vi "ExTestKineticsVClk.vi"() -> ()   [LabVIEW 2010]
panel:
  out "Max Vertical Clock":u32
  out "Min Vertical Clock":u32
  out "Vertical Clock":u32
  in  "Vertical Clock":u32=2 min=1 max=16 step=1
  in  "Enum":T1(ring)
  in  "Window Size":u32=10 min=1 step=1
  out "Boolean":bool
  out "x Size":u32
  out "x post":u32
  out "x pre":u32
  out "y Size":u32
  out "y post":u32
  out "y pre":u32
  in  "Software Accumulation":u32=1 min=1 step=1
  in  "Intensifier":bool
  in  "Temperature":dbl=-10.0 format="%.2f"
  in  "Exposure":dbl min=0.0 step=1e-06 format="%.5f"
  in  "stop":bool
  in  "Store":bool
  out "error out":errorcluster
  in  "error in (no error)":errorcluster
  # "ExCircularBufBin2x:\nThis example only works with cameras with circualar \nbuffer capability. This routine will continously display an\nimage binned by 2 in both the x and the y direction. It \nwill store in append mode the frames while \nthe store toggle switch is on."
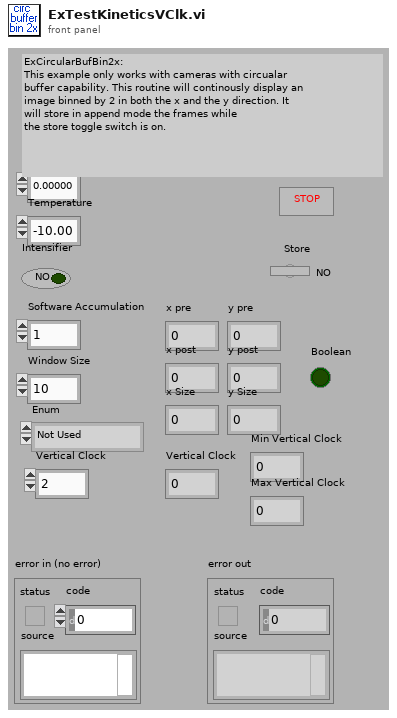
[diagram p1: front panel]
types:
  T1 = enum32{"Not Used", "No Trigger", "Single Trigger", "Multiple Trigger"}
  T2 = cluster{"Param ID":u32, "Avail Flag":u8, "Current Value":dbl, "Default Value":dbl, "Min Value":dbl, "Max Value":dbl, "Increment":dbl, "Data Type":u32, "Access Type":u32, "Bit Used Flag":u32, "Number of Enums":u32, "Description":string}
  T3 = cluster{"Pre Y":u32, "Post Y":u32, "Parallel (Y) Size":u32, "Pre X":u32, "Post X":u32, "Serial (X) Size":u32}
  T4 = cluster{"Camera Handle":u32, "Pulser Handle":u32, "File Handle":u32, "Display Handle":u32, "Image Handle":u32}
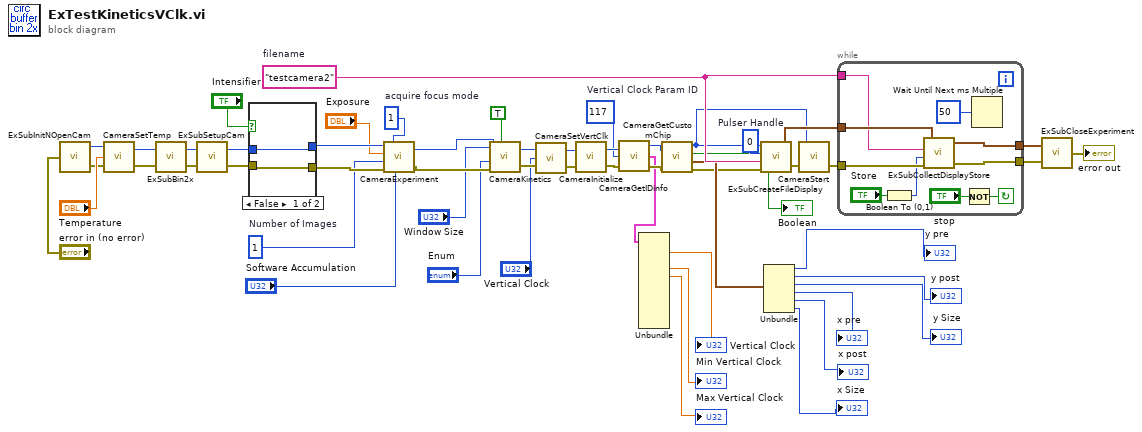
[diagram p0: block diagram]
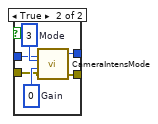
[diagram p2: hidden frame]
diagram:
  w5 = 117  # Vertical Clock Param ID
  w45 = u32 0  # Pulser Handle
  w21 = u32 1  # acquire focus mode
  w23 = u32 1  # Number of Images
  w54 = "testcamera2"  # filename
  n1 = call "ExSubInitNOpenCam.vi"("error in (no error)"="error in (no error)") -> ("Camera Handle"=w43:u32, "error out"=w41:errorcluster)
  n2 = call <userlib>:"CameraSetTemp.vi"("error in (no error)"=w41, "Temperature"="Temperature", "Camera Handle"=w43) -> ("error out"=w29:errorcluster, "Camera Handle"=w30:u32)
  n3 = call "ExSubBin2x.vi"("error in (no error)"=w29, "Camera Handle"=w30) -> ("error out"=w40:errorcluster, "Camera Handle"=w46:u32)
  n4 = call "ExSubSetupCam.vi"("error in (no error)"=w40, "Camera Handle"=w46) -> ("error out"=w27:errorcluster, "Camera Handle"=w28:u32)
  n5 = case shown="False" "Intensifier" {
    tunnel: [w56 w62] -> w26
    tunnel: [w55 w61] -> w25
    tunnel: w28 -> [w56 w58]
    tunnel: w27 -> [w55 w57]
    frame False {
    }
    frame True {
      w59 = u32 0  # Gain
      w60 = u32 3  # Mode
      n6 = call <userlib>:"CameraIntensMode.vi"("error in"=w57, "Intensifier Gain"=w59, "Mode"=w60, "Camera Handle"=w58) -> ("error out"=w61:errorcluster, "Camera Handle"=w62:u32)
    }
  }
  n7 = call <userlib>:"CameraExperiment.vi"("Number of Accumulations"="Software Accumulation", "Acquire / Focus Flag"=w21, "error in"=w25, "Number of Images"=w23, "Exposure (sec)"="Exposure", "Camera Handle"=w26) -> ("error out"=w19:errorcluster, "Camera Handle"=w20:u32)
  n8 = call <userlib>:"CameraKinetics.vi"("Camera Handle"=w20, "Window Size"="Window Size", "TriggerMode"="Enum", "error in (no error)"=w19, "Enable/Disable Kinetics"=TRUE) -> ("Camera Handle"=w13:u32, "error out"=w14:errorcluster)
  n9 = call <userlib>:"CameraSetVertClk.vi"("error in (no error)"=w14, "Vertical Clock"="Vertical Clock", "Camera Handle"=w13) -> ("error out"=w11:errorcluster, "Camera Handle"=w10:u32)
  n10 = call <userlib>:"CameraInitialize.vi"("error in"=w11, "Camera Handle"=w10) -> ("error out"=w9:errorcluster, "Camera Handle"=w6:u32)
  n11 = call <userlib>:"CameraGetIDinfo.vi"("error in"=w9, "Param ID"=w5, "Camera handle"=w6) -> ("error out"=w8:errorcluster, "Param ID Information"=w4:T2, "Camera handle"=w7:u32)
  n12 = Unbundle(w4) -> ("Current Value"=→"Vertical Clock":dbl, "Min Value"=→"Min Vertical Clock":dbl, "Max Value"=→"Max Vertical Clock":dbl)  [unwired: 9 out]
  n13 = call <userlib>:"CameraGetCustomChip.vi"("Camera Handle"=w7, "error in (no error)"=w8) -> ("Camera Handle"=w16:u32, "Custum chip Enable/Disable status"=→"Boolean":bool, "CameraGetCustomChip"=w39:T3, "error out"=w32:errorcluster)
  n14 = call "ExSubCreateFileDisplay.vi"("error in (no error)"=w32, "File and Display Name"=w54, "Pulser Handle"=w45, "Camera Handle"=w16) -> ("error out"=w47:errorcluster, "Handles Out"=w52:T4)
  n15 = Unbundle(w39) -> ("Pre Y"=→"y pre":u32, "Post Y"=→"y post":u32, "Parallel (Y) Size"=→"y Size":u32, "Pre X"=→"x pre":u32, "Post X"=→"x post":u32, "Serial (X) Size"=→"x Size":u32)
  n16 = call <userlib>:"CameraStart.vi"("error in"=w47, "Camera Handle"=w16) -> ("error out"=w48:errorcluster)  [unwired: 1 out]
  n17 = while {
    tunnel: w52 -> [w71]
    tunnel: w48 -> [w70]
    tunnel: w54 -> [w63]
    tunnel: [w68] -> w50
    tunnel: [w69] -> w51
    stop <- w66 continue-if-true
    n18 = Boolean To (0,1)(Boolean="Store") -> (0, 1=w64:i16)
    n19 = call "ExSubCollectDisplayStore.vi"("error in (no error)"=w70, "Store flag"=w64, "Display Title"=w63, "Handle Cluster"=w71) -> ("error out"=w68:errorcluster, "Handle Cluster Out"=w69:T4)  [unwired: 1 out]
    n20 = Not(x="stop") -> (.not. x?=w66:bool)
    n21 = Wait Until Next ms Multiple(millisecond multiple=u32 50) -> ()  [unwired: 1 out]
  }
  n22 = call "ExSubCloseExperiment.vi"("error in (no error)"=w50, "Handles In"=w51) -> ("error out"=→"error out":errorcluster)
